vi "rad_Retrieve Application Image From Target.vi"(7 "App Images Temp Folder":path=path "C:/dev/Architectures/Reference Designs/Application Deployment and Replication/Application Deployment Utility/trunk/source/Application Images/_temp", 8 "error in (no error)":errorcluster, 10 "Target settings":T1={"Hostname"="", "Serial number"="", "Product name"="", "Product code"=0, "System status"="", "Credential type"=enum."None/Unlocked", "User added?"=FALSE, "Primary NIC"={"MAC address"="", "IP Address Request Mode"=2, "IP address"="", "Subnet mask"="", "Gateway"="", "DNS server"=""}} {"Primary NIC"."IP Address Request Mode" items=["Static"=1, "DHCP/Link-Local"=2, "Link-Local Only"=4, "DHCP Only"=8]}, 11 "App Images Folder":path) -> (0 "error out":errorcluster, 2 "Cancelled":bool, 3 "New App Image Path":path)   [LabVIEW 2014]
uses:
  TypeDefs/rad_Application Image Properties.ctl
  TypeDefs/rad_FPGA Properties.ctl
  TypeDefs/rad_FPGA Flash Properties.ctl
  Targets/TypeDefs/rad_Target Information.ctl
  Targets/TypeDefs/rad_Target Network Settings.ctl
  TypeDefs/rad_Retrieve Application Image States.ctl
  TypeDefs/rad_App Images Settings.ctl
  TypeDefs/rad_Deployment Status Data Type.ctl
  TypeDefs/rad_Deployment Progress Data Type.ctl
  TypeDefs/rad_Deployment Notifiers.ctl
panel:
  in  "State Data":T6
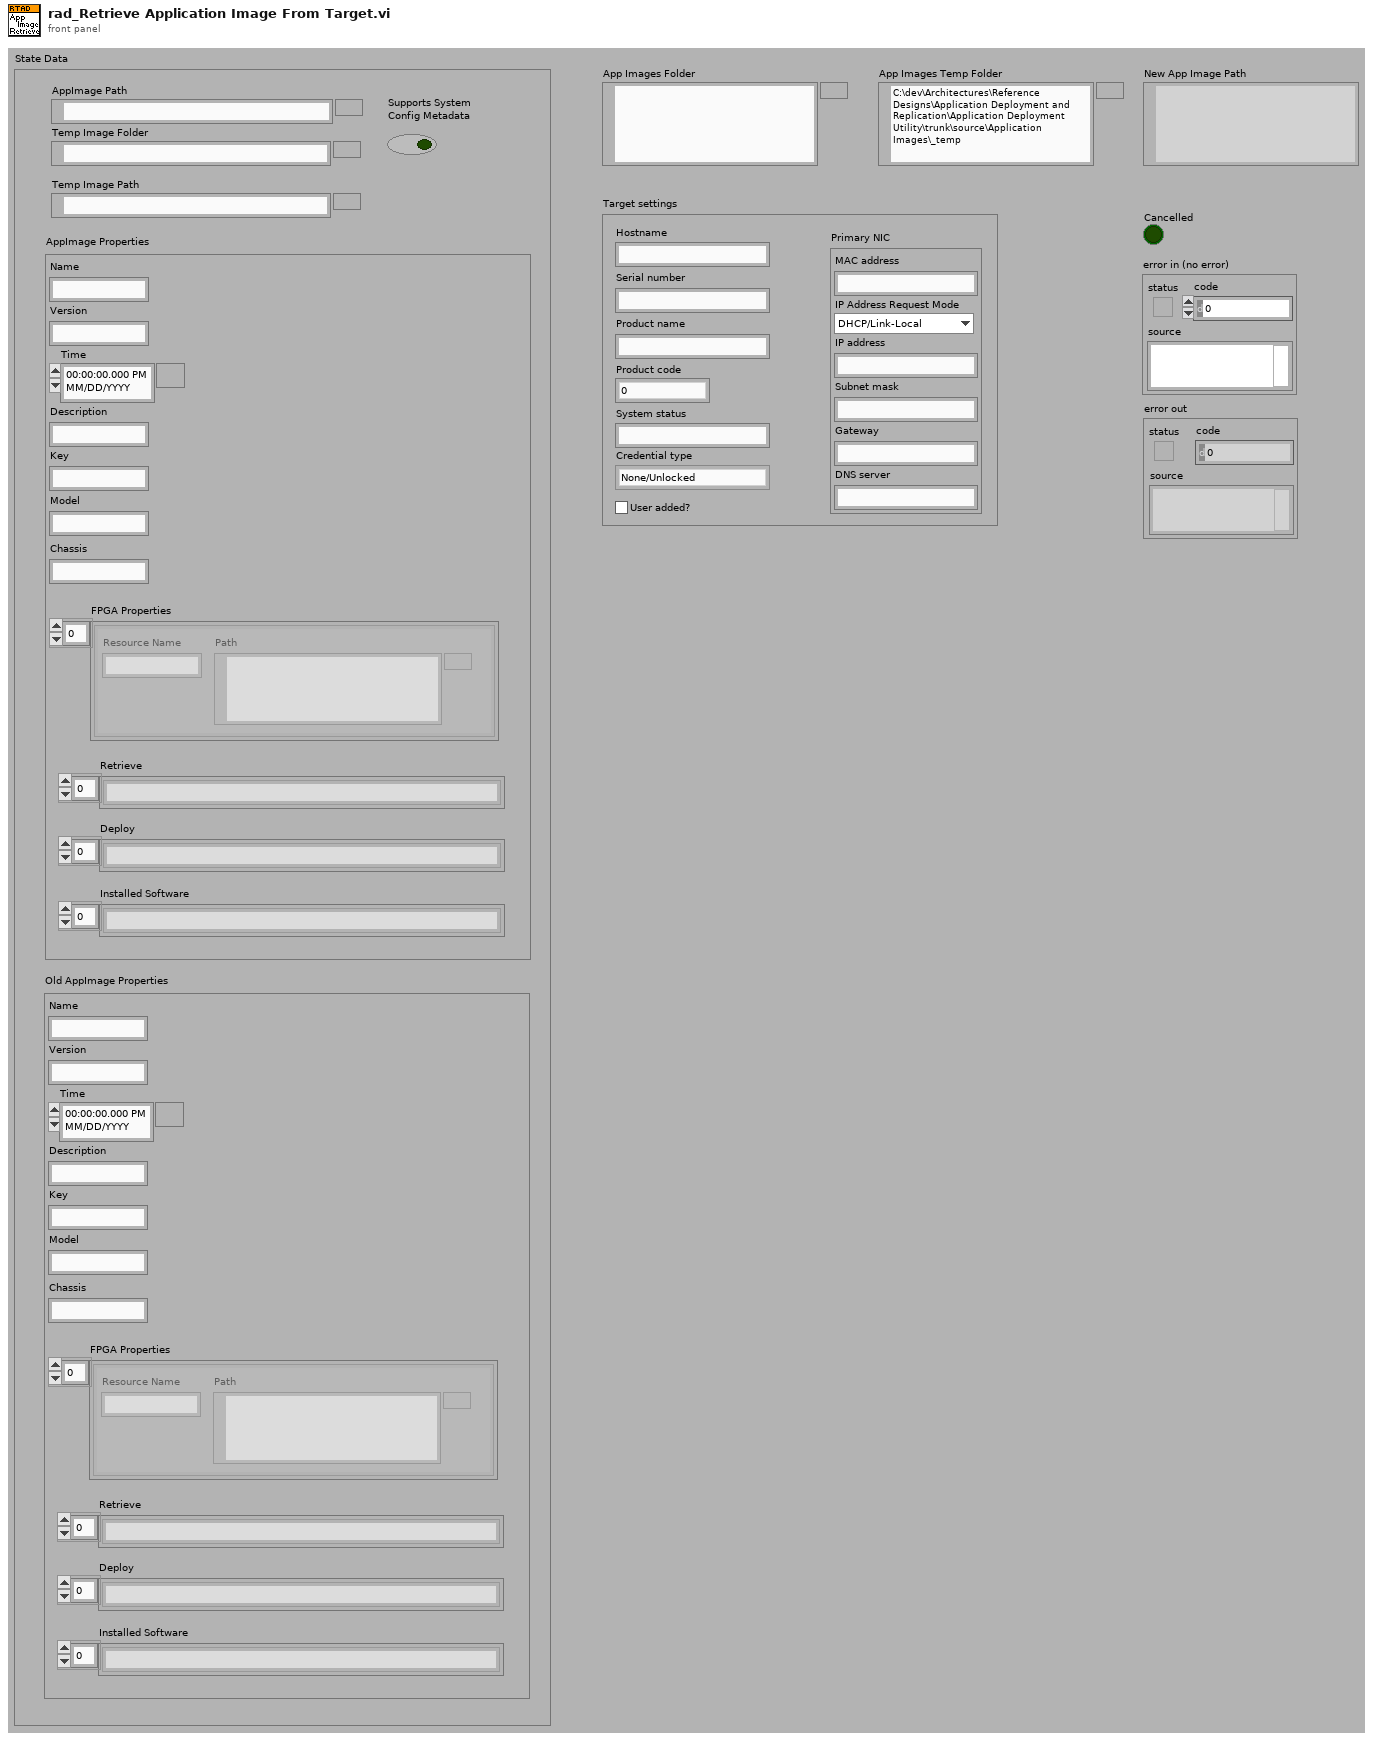
[diagram p1: front panel]
types:
  T1 = typedef "rad_Target Information.ctl" = cluster{"Hostname":string, "Serial number":string, "Product name":string, "Product code":i32, "System status":string, "Credential type":enum16{"None/Unlocked", "FTP Password", "NIAuth Credentials"}, "User added?":bool, "Primary NIC":T2}
  T2 = typedef "rad_Target Network Settings.ctl" = cluster{"MAC address":string, "IP Address Request Mode":i32, "IP address":string, "Subnet mask":string, "Gateway":string, "DNS server":string}
  T3 = typedef "rad_Application Image Properties.ctl" = cluster{"Name":string, "Version":string, "Time":timestamp, "Description":string, "Key":string, "Chassis":string, "FPGA Properties":T4, "Model":string, "Retrieve":string[], "Deploy":string[], "Installed Software":string[]}
  T4 = typedef "rad_FPGA Properties.ctl" = T5[]
  T5 = typedef "rad_FPGA Flash Properties.ctl" = cluster{"Resource Name":string, "Path":path}
  T6 = cluster{"AppImage Path":path, "Temp Image Folder":path, "AppImage Properties":T3, "App Image Info File Path":path, "New Image?":bool, "Selected Existing Image":path, "Bitfiles Modified?":bool, "Old AppImage Properties":T3, "Temp Image Path":path, "Supports System\nConfig Metadata":bool}
  T7 = typedef "rad_Retrieve Application Image States.ctl" = enum16{"Verify App Image Directory", "Get Target's Image Info", "Select Image Prop. Source", "Find Existing Disk Image", "Get Disk Image Properties", "Create New Image", "Set Image Properties", "Get Image Save Location", "GetInstalledSoftware", "Create App Image Info File", "Deploy New Files to Target", "Retrieve Application Image", "PackageImage", "Cleanup", "Exit"}
  T8 = typedef "rad_App Images Settings.ctl" = cluster{"App Images Folder":path, "App Images Temp Folder":path, "CurrentVersion":string}
  T9 = enum16{"None/Unlocked", "FTP Password", "NIAuth Credentials"}
  T10 = typedef "rad_Deployment Notifiers.ctl" = cluster{"Status":refnum<notifier>, "Progress":refnum<notifier>}
  T11 = typedef "rad_Deployment Progress Data Type.ctl" = i8
  T12 = typedef "rad_Deployment Status Data Type.ctl" = string
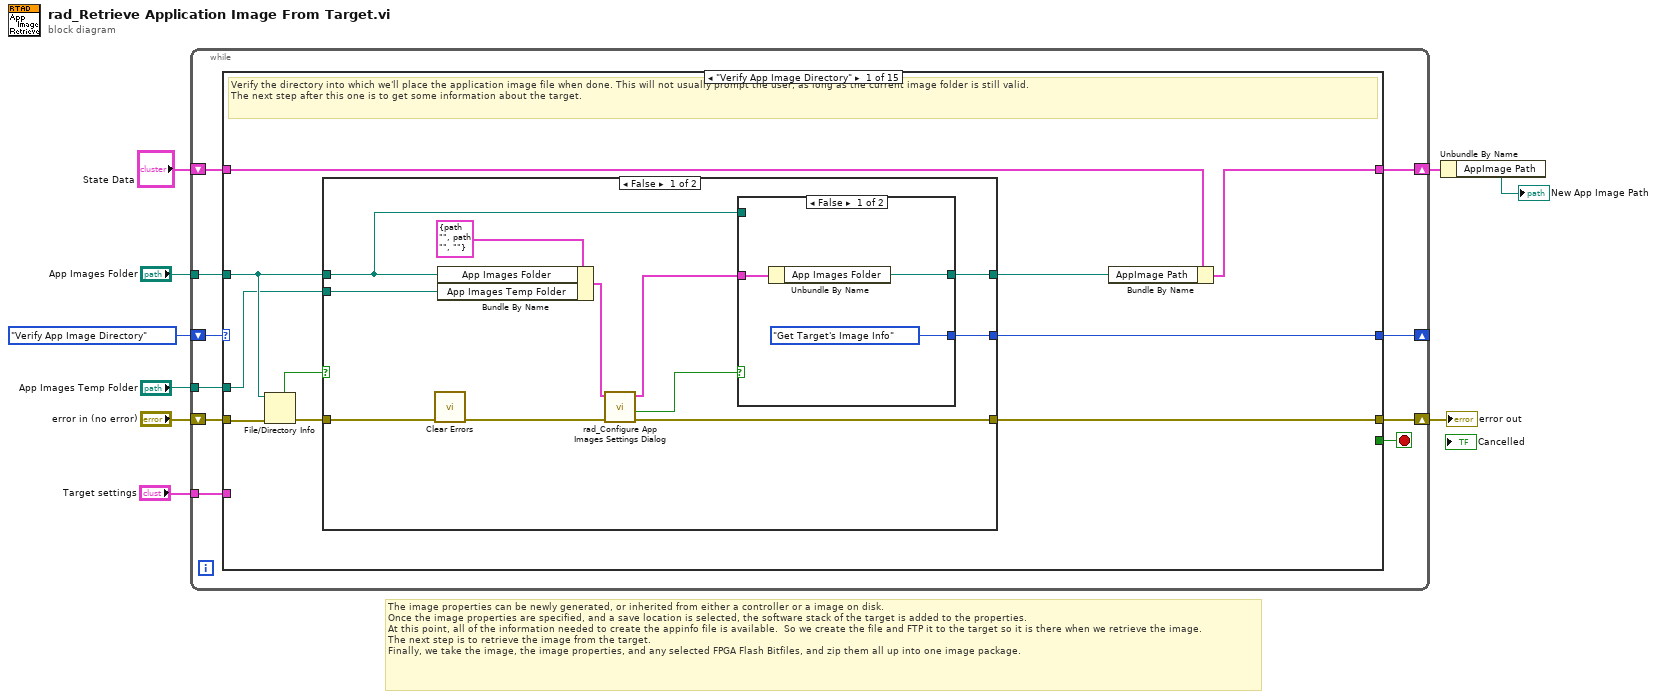
[diagram p0: block diagram]
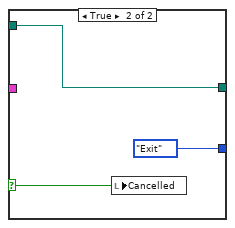
[diagram p2: hidden frame]
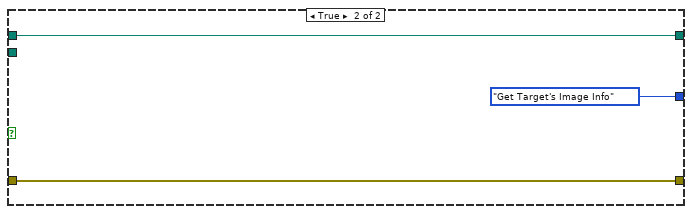
[diagram p3: hidden frame]
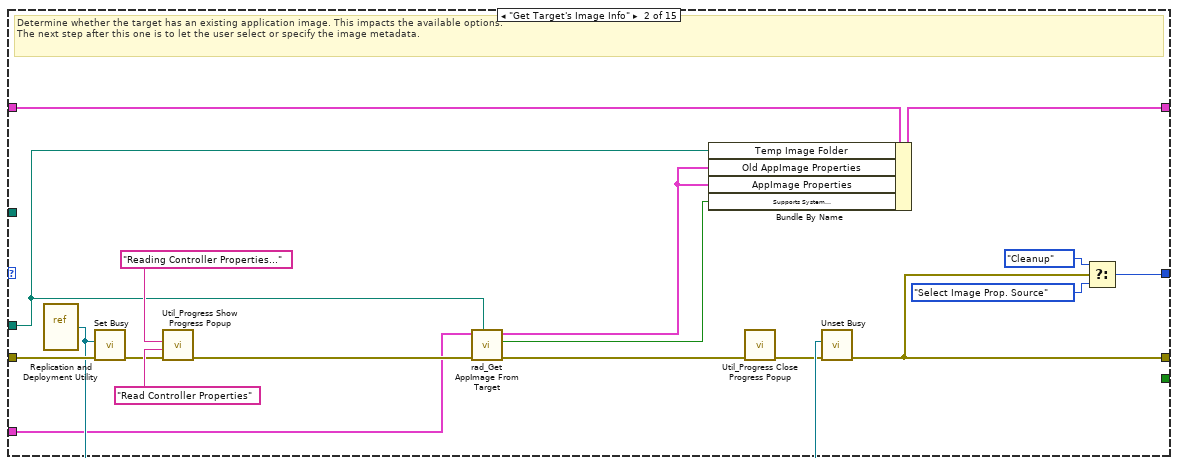
[diagram p4: hidden frame]
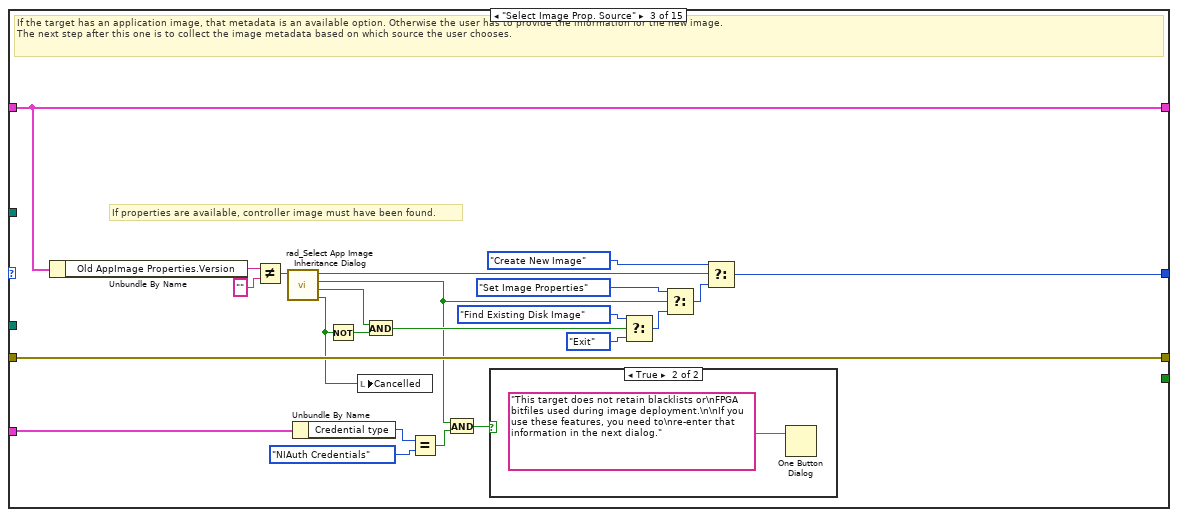
[diagram p5: hidden frame]
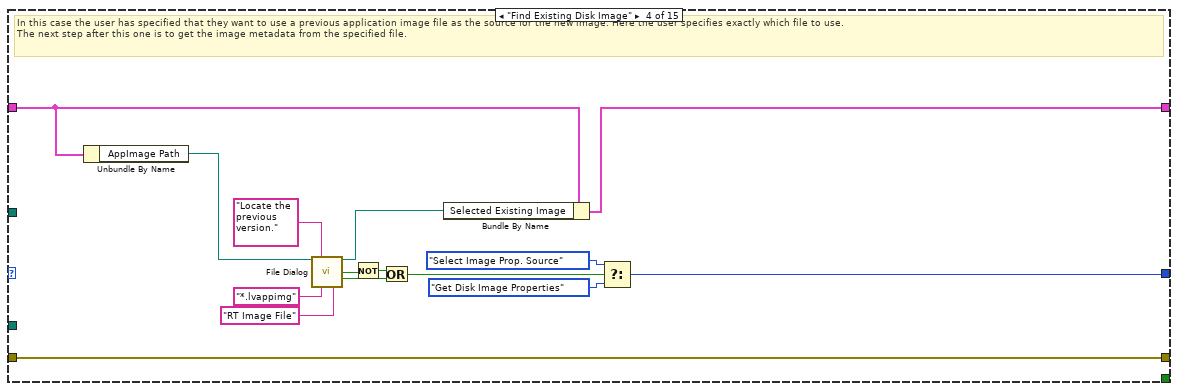
[diagram p7: hidden frame]
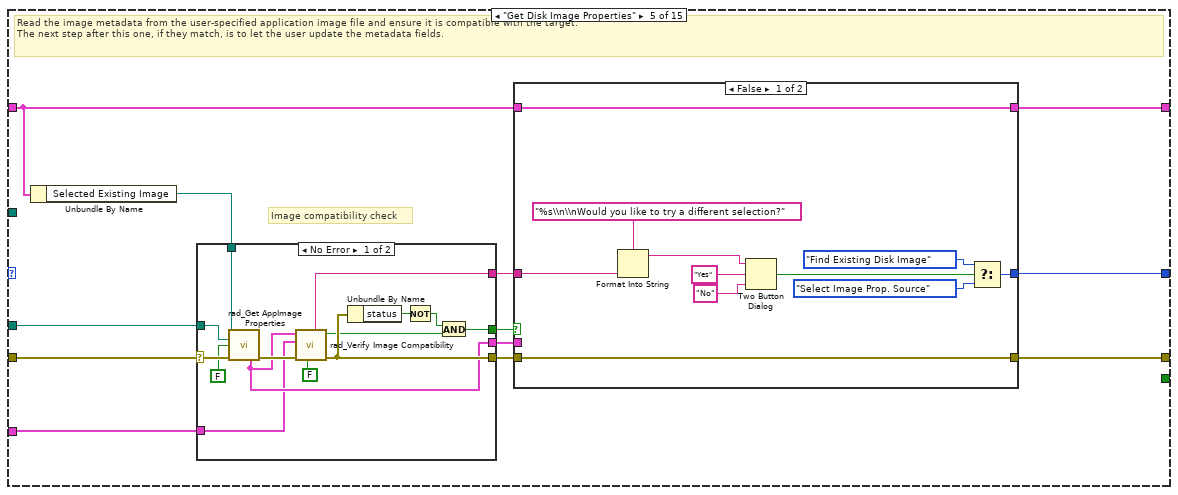
[diagram p8: hidden frame]
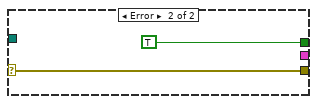
[diagram p9: hidden frame]
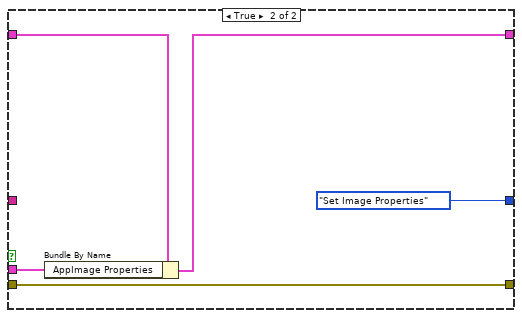
[diagram p10: hidden frame]
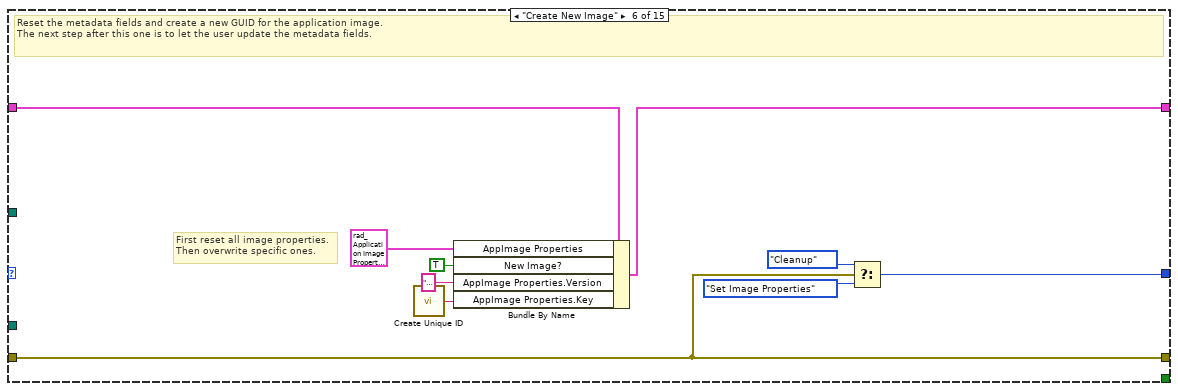
[diagram p11: hidden frame]
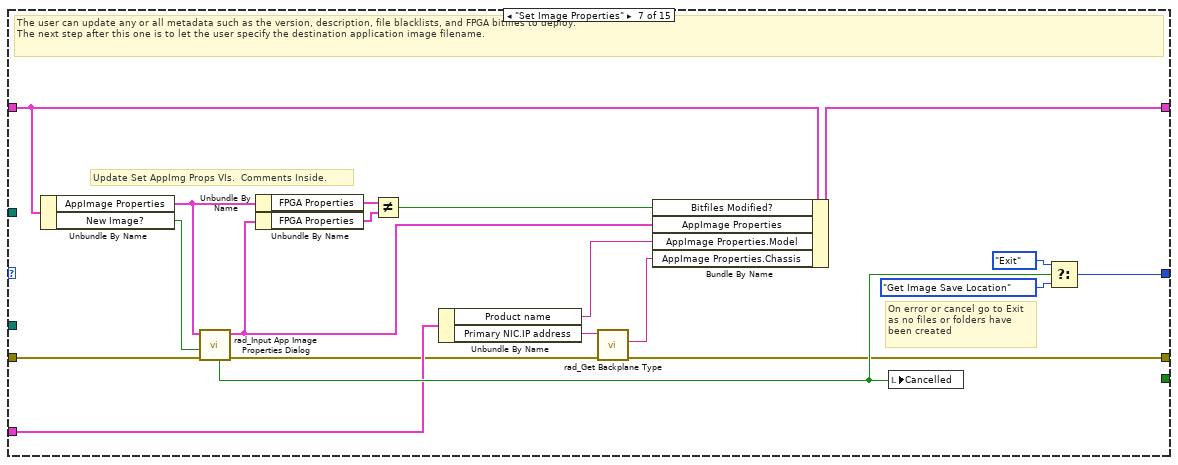
[diagram p12: hidden frame]
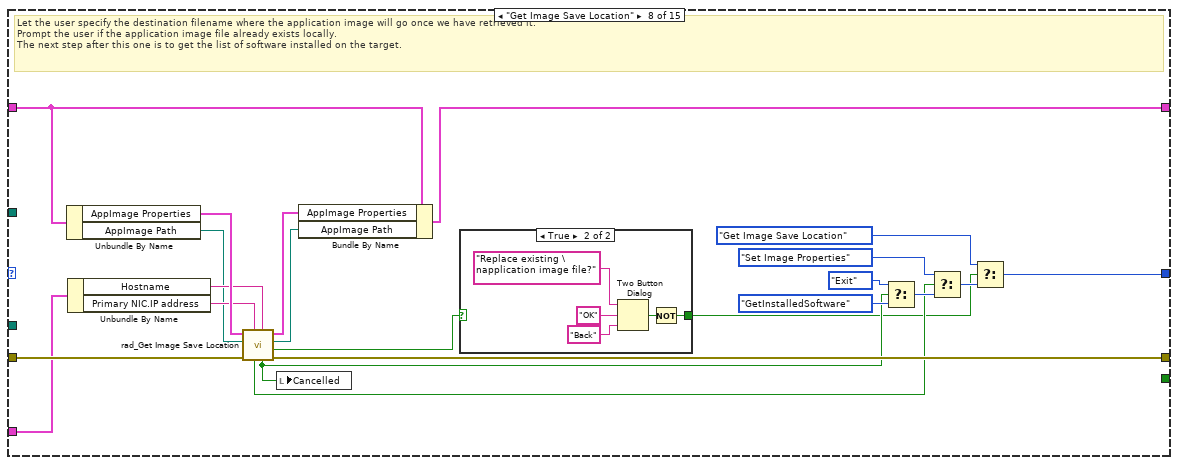
[diagram p13: hidden frame]
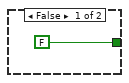
[diagram p14: hidden frame]
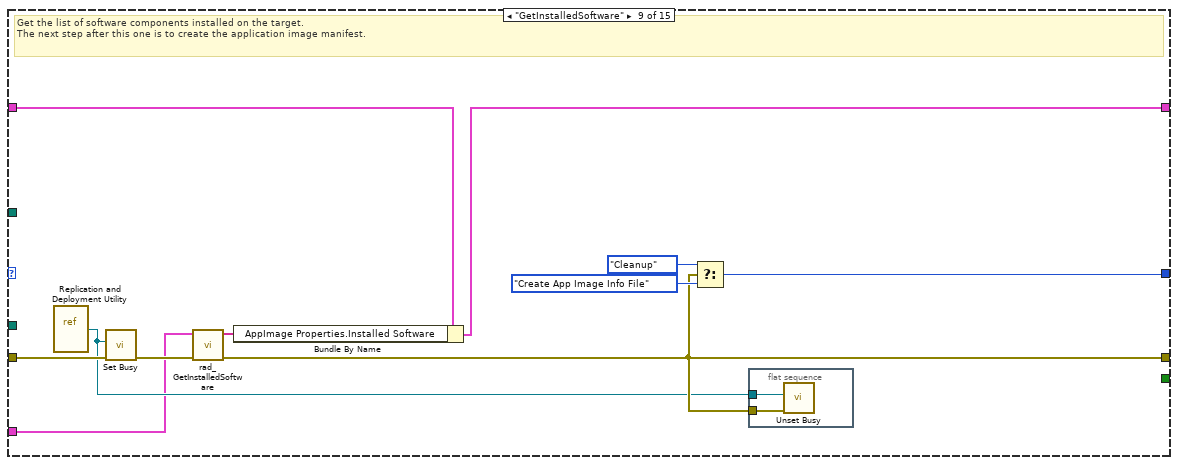
[diagram p15: hidden frame]
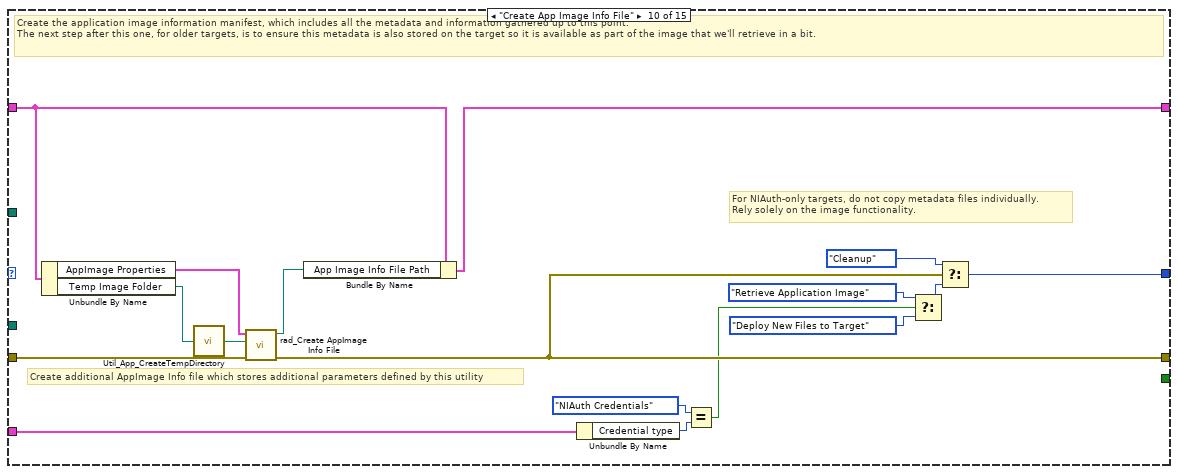
[diagram p16: hidden frame]
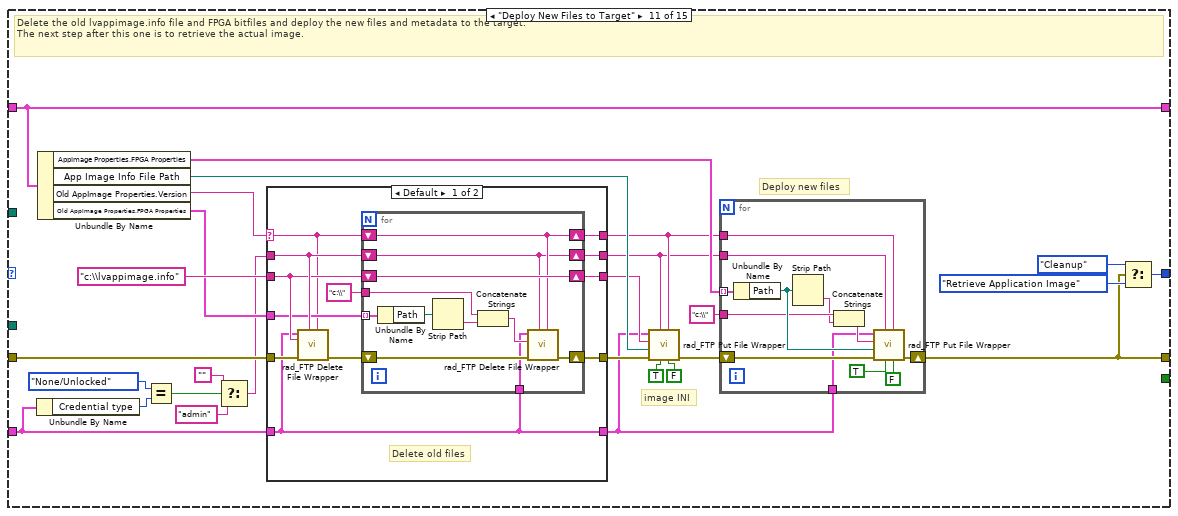
[diagram p17: hidden frame]
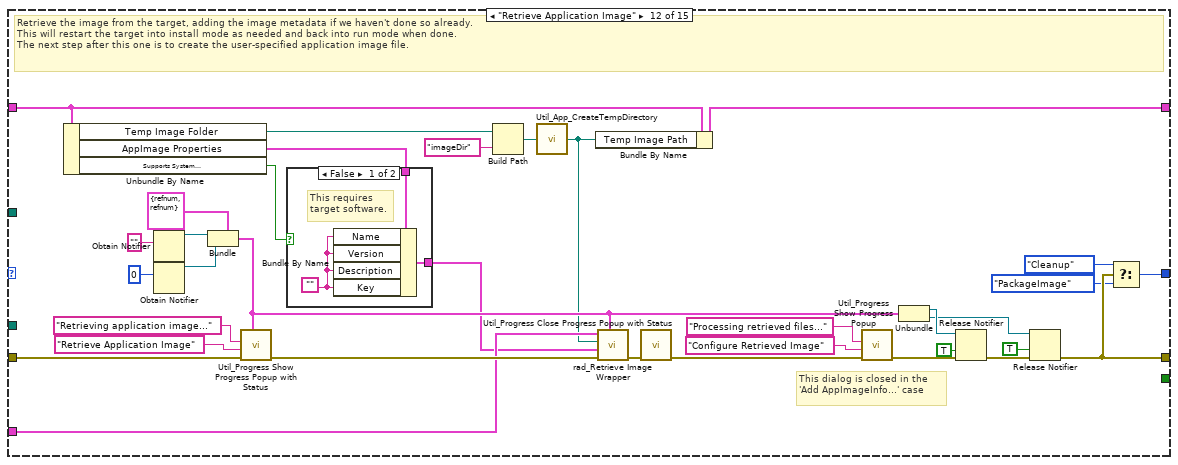
[diagram p19: hidden frame]
diagram:
  # "The image properties can be newly generated, or inherited from either a controller or a image on disk.\nOnce the image properties are specified, and a save location is selected, the software stack of the target is added to the properties.\nAt this point, all of the information needed to create the appinfo file is available.  So we create the file and FTP it to the target so it is there when we retrieve the image.\nThe next step is to retrieve the image from the target.\nFinally, we take the image, the image properties, and any selected FPGA Flash Bitfiles, and zip them all up into one image package."
  n1 = while {
    shift-right: [w18] -> _
    shift-left: rad_Retrieve_Application_Image_States."Verify App Image Directory" ("Retrieve App Images States") -> [w19]
    shift-right: [w15] -> w5
    shift-left: "State Data" -> [w16]
    shift-right: [w13] -> w6
    shift-left: "error in (no error)" -> [w14]
    tunnel: "App Images Folder" -> [w12]
    tunnel: "App Images Temp Folder" -> [w11]
    tunnel: "Target settings" -> [w10]
    stop <- w17 stop-if-true
    n2 = case shown="\"Verify App Image Directory\"" w19 {
      tunnel: [w23 w66 w78 w105 w117 w157 w179 w185 w214 w237 w249 w337 rad_Retrieve_Application_Image_States."Cleanup" ("Retrieve App Images States") rad_Retrieve_Application_Image_States."Exit" ("Retrieve App Images States") _] -> w18
      tunnel: [_ _ _ _ _ _ _ _ _ _ _ _ _ _ TRUE] -> w17
      tunnel: w16 -> [w22 w61 w90 w93 w114 w153 w174 w199 w217 w232 w264 w335 w347 w357 w371]
      tunnel: [w21 w65 w90 w104 w110 w160 w175 w198 w216 w234 w264 w336 w347 w357 w371] -> w15
      tunnel: w14 -> [w29 w60 w79 w106 w116 w151 w178 w201 w211 w230 w254 w330 w349 w351 w374]
      tunnel: [w26 w58 w79 w106 w112 w151 w161 w194 w212 w235 w248 w318 w348 w353 w374] -> w13
      tunnel: w12 -> [w25 _ _ _ _ _ _ _ _ _ _ _ _ _ _]
      tunnel: w11 -> [w24 w51 _ _ w111 _ _ _ _ _ _ _ _ _ _]
      tunnel: w10 -> [_ w52 w73 _ w107 _ w163 w183 w208 w224 w245 w311 _ _ _]
      frame "Verify App Image Directory" {
        # "Verify the directory into which we'll place the application image file when done. This will not usually prompt the user, as long as the current image folder is still valid.\nThe next step after this one is to get some information about the target."
        n3 = File/Directory Info(path=w25, error in=w29) -> (directory=w28:bool, error out=w27:errorcluster)  [unwired: 5 out]
        n4 = case shown="False" w28 {
          tunnel: w27 -> [w40 w49]
          tunnel: [w38 w49] -> w26
          tunnel: w25 -> [w30 w47]
          tunnel: w24 -> [w39 _]
          tunnel: [w35 rad_Retrieve_Application_Image_States."Get Target's Image Info" ("Retrieve App Images States")] -> w23
          tunnel: [w31 w47] -> w20
          frame False {
            n5 = call <vilib>:"Clear Errors.vi"("error in (no error)"=w40) -> ("error out"=w32:errorcluster)  [unwired: 5 in, 1 out]
            n6 = Bundle By Name(cluster=T8 {"App Images Folder"=path "", "App Images Temp Folder"=path "", "CurrentVersion"=""} ("App Images Settings"), "App Images Folder"=w30, "App Images Temp Folder"=w39) -> (w33:T8)
            n7 = call "rad_Configure App Images Settings Dialog.vi"("error in (no error)"=w32, "App Images Settings"=w33) -> ("error out"=w38:errorcluster, "Cancelled"=w37:bool, "App Images Settings"=w36:T8)  [unwired: 7 out]
            n8 = case shown="False" w37 {
              selector: w37 -> [_ w44]
              tunnel: w36 -> [w42 _]
              tunnel: [rad_Retrieve_Application_Image_States."Get Target's Image Info" ("Retrieve App Images States") rad_Retrieve_Application_Image_States."Exit" ("Retrieve App Images States")] -> w35
              tunnel: [w41 w45] -> w31
              tunnel: w30 -> [_ w45]
              frame False {
                n9 = Unbundle By Name(w42) -> ("App Images Folder"=w41:path)
              }
              frame True {
                n10 = local write "Cancelled"(w44) -> ()
              }
            }
          }
          frame True {
          }
        }
        n11 = Bundle By Name(cluster=w22, "AppImage Path"=w20) -> (w21:T6)
      }
      frame "Get Target's Image Info" {
        # "Determine whether the target has an existing application image. This impacts the available options.\nThe next step after this one is to let the user select or specify the image metadata."
        n12 = vi-ref "Replication and Deployment Utility.vi"() -> (w57:refnum<vi>)
        n13 = call <vilib>:"Set Busy.vi"("error in (no error)"=w60, "VI reference (current VI)"=w57) -> ("error out"=w59:errorcluster)  [unwired: 8 in, 1 out]
        n14 = call "Util_Progress Show Progress Popup.vi"("error in (no error)"=w59, "Title"="Read Controller Properties", "Message"="Reading Controller Properties...") -> ("error out"=w55:errorcluster)  [unwired: 8 in]
        n15 = call "rad_Get AppImage From Target.vi"("Temp Folder"=w51, "error in (no error)"=w55, "Target settings"=w52) -> ("error out"=w54:errorcluster, "Supports System\nConfig Metadata"=w50:bool, "AppImage Properties"=w53:T3)  [unwired: 6 in]
        n16 = Bundle By Name(cluster=w61, "Temp Image Folder"=w51, "Old AppImage Properties"=w53, "AppImage Properties"=w53, "Supports System\nConfig Metadata"=w50) -> (w65:T6)
        n17 = call "Util_Progress Close Progress Popup.vi"("error in (no error)"=w54) -> ("error out"=w56:errorcluster)  [unwired: 10 in]
        n18 = call <vilib>:"Unset Busy.vi"("error in (no error)"=w56, "VI reference (current VI)"=w57) -> ("error out"=w58:errorcluster)  [unwired: 9 in]
        n19 = Select(t=rad_Retrieve_Application_Image_States."Cleanup", s=w58, f=rad_Retrieve_Application_Image_States."Select Image Prop. Source" ("Retrieve App Images States")) -> (s? t:f=w66:T7)
      }
      frame "Select Image Prop. Source" {
        # "If properties are available, controller image must have been found."
        # "If the target has an application image, that metadata is an available option. Otherwise the user has to provide the information for the new image.\nThe next step after this one is to collect the image metadata based on which source the user chooses."
        n20 = Unbundle By Name(w90) -> ("Old AppImage Properties.Version"=w89:string)
        n21 = Not Equal?(x=w89, y="") -> (x != y?=w87:bool)
        n22 = call "rad_Select App Image Inheritance Dialog.vi"("Controller Image Available?"=w87) -> ("Cancel"=w74:bool, "Disc Image"=w77:bool, "Controller Image"=w69:bool, "New Image"=w86:bool)  [unwired: 7 in]
        n23 = Unbundle By Name(w73) -> ("Credential type"=w72:T9)
        n24 = Not(x=w74) -> (.not. x?=w76:bool)
        n25 = local write "Cancelled"(w74) -> ()
        n26 = And(x=w77, y=w76) -> (x .and. y?=w75:bool)
        n27 = Equal?(x=w72, y=T9."NIAuth Credentials" ("Credential type")) -> (x = y?=w70:bool)
        n28 = And(x=w69, y=w70) -> (x .and. y?=w68:bool)
        n29 = case shown="True" w68 {
          frame False {
          }
          frame True {
            n30 = One Button Dialog(message="This target does not retain blacklists or\nFPGA bitfiles used during image deployment.\n\nIf you use these features, you need to\nre-enter that information in the next dialog.") -> ()  [unwired: 1 in, 1 out]
          }
        }
        n31 = Select(t=rad_Retrieve_Application_Image_States."Find Existing Disk Image" ("Retrieve App Images States"), s=w75, f=rad_Retrieve_Application_Image_States."Exit" ("Retrieve App Images States")) -> (s? t:f=w81:T7)
        n32 = Select(t=rad_Retrieve_Application_Image_States."Set Image Properties" ("Retrieve App Images States"), s=w69, f=w81) -> (s? t:f=w83:T7)
        n33 = Select(t=rad_Retrieve_Application_Image_States."Create New Image" ("Retrieve App Images States"), s=w86, f=w83) -> (s? t:f=w78:T7)
      }
      frame "Find Existing Disk Image" {
        # "In this case the user has specified that they want to use a previous application image file as the source for the new image. Here the user specifies exactly which file to use.\nThe next step after this one is to get the image metadata from the specified file."
        n34 = Unbundle By Name(w93) -> ("AppImage Path"=w92:path)
        n35 = call "File Dialog"("start path"=w92, "prompt"="Locate the previous version.", "pattern (all files)"="*.lvappimg", "pattern label"="RT Image File") -> ("selected path"=w94:path, "exists"=w101:bool, "cancelled"=w99:bool)  [unwired: 8 in, 1 out]
        n36 = Not(x=w101) -> (.not. x?=w100:bool)
        n37 = Or(x=w100, y=w99) -> (x .or. y?=w97:bool)
        n38 = Bundle By Name(cluster=w93, "Selected Existing Image"=w94) -> (w104:T6)
        n39 = Select(t=rad_Retrieve_Application_Image_States."Select Image Prop. Source" ("f"), s=w97, f=rad_Retrieve_Application_Image_States."Get Disk Image Properties") -> (s? t:f=w105:T7)
      }
      frame "Get Disk Image Properties" {
        # "Image compatibility check"
        # "Read the image metadata from the user-specified application image file and ensure it is compatible with the target.\nThe next step after this one, if they match, is to let the user update the metadata fields."
        n40 = Unbundle By Name(w114) -> ("Selected Existing Image"=w118:path)
        n41 = case shown="No Error" w116 {
          selector: w116 -> [w124 w134]
          tunnel: w111 -> [w125 _]
          tunnel: w118 -> [w126 _]
          tunnel: [w132 w134] -> w113
          tunnel: [w130 TRUE] -> w115
          tunnel: [w121 _] -> w109
          tunnel: w107 -> [w120 _]
          tunnel: [w119 _] -> w108
          frame No Error {
            n42 = call "rad_Get AppImage Properties.vi"("AppImage Path"=w126, "App Image Temp Folder"=w125, "Show FP"=FALSE, "error in (no error)"=w124) -> ("AppImage Properties"=w121:T3, "error out"=w123:errorcluster)  [unwired: 5 in, 5 out]
            n43 = call "rad_Verify Image Compatibility.vi"("Require Identical Chassis?"=FALSE, "error in (no error)"=w123, "Target address"=w120, "AppImage Properties"=w121) -> ("error out"=w132:errorcluster, "Compatible?"=w129:bool, "Status message"=w119:string)  [unwired: 5 in]
            n44 = Unbundle By Name(w132) -> ("status"=w131:bool)
            n45 = Not(x=w131) -> (.not. x?=w128:bool)
            n46 = And(x=w128, y=w129) -> (x .and. y?=w130:bool)
          }
          frame Error {
          }
        }
        n47 = case shown="False" w115 {
          tunnel: [w140 rad_Retrieve_Application_Image_States."Set Image Properties" ("Retrieve App Images States")] -> w117
          tunnel: w114 -> [w138 w150]
          tunnel: w113 -> [w139 w146]
          tunnel: [w139 w146] -> w112
          tunnel: [w138 w148] -> w110
          tunnel: w109 -> [_ w147]
          tunnel: w108 -> [w136 _]
          frame False {
            n48 = Format Into String(format string="%s\\n\\nWould you like to try a different selection?" ("message"), w136) -> (resulting string=w135:string)  [unwired: 2 in, 1 out]
            n49 = Two Button Dialog(message=w135, 1:"No" ("F button name (\"Cancel\")"), 2:"Yes" ("T button name (\"OK\")")) -> (T button?=w142:bool)
            n50 = Select(t=rad_Retrieve_Application_Image_States."Find Existing Disk Image" ("Retrieve App Images States"), s=w142, f=rad_Retrieve_Application_Image_States."Select Image Prop. Source" ("Retrieve App Images States")) -> (s? t:f=w140:T7)
          }
          frame True {
            n51 = Bundle By Name(cluster=w150, "AppImage Properties"=w147) -> (w148:T6)
          }
        }
      }
      frame "Create New Image" {
        # "First reset all image properties.\nThen overwrite specific ones."
        # "Reset the metadata fields and create a new GUID for the application image.\nThe next step after this one is to let the user update the metadata fields."
        n52 = call "Create Unique ID.vi"() -> ("ID String"=w156:string)  [unwired: 1 in]
        n53 = Bundle By Name(cluster=w153, "AppImage Properties"=T3 {"Name"="", "Version"="", "Time"=timestamp(0 s since 1904-01-01), "Description"="", "Key"="", "Chassis"="", "FPGA Properties"=[], "Model"="", "Retrieve"=[], "Deploy"=[], "Installed Software"=[]}, "New Image?"=TRUE, "AppImage Properties.Version"="1.0.0", "AppImage Properties.Key"=w156) -> (w160:T6)
        n54 = Select(t=rad_Retrieve_Application_Image_States."Cleanup", s=w151, f=rad_Retrieve_Application_Image_States."Set Image Properties" ("Retrieve App Images States")) -> (s? t:f=w157:T7)
      }
      frame "Set Image Properties" {
        # "Update Set AppImg Props VIs.  Comments Inside."
        # "On error or cancel go to Exit\nas no files or folders have\nbeen created"
        # "The user can update any or all metadata such as the version, description, file blacklists, and FPGA bitfiles to deploy.\nThe next step after this one is to let the user specify the destination application image filename."
        n55 = Unbundle By Name(w174) -> ("AppImage Properties"=w169:T3, "New Image?"=w170:bool)
        n56 = call "rad_Input App Image Properties Dialog.vi"("error in (no error)"=w178, "New Image?"=w170, "AppImage Properties"=w169) -> ("error out"=w162:errorcluster, "AppImage Properties"=w167:T3, "Cancelled"=w168:bool)  [unwired: 4 in, 2 out]
        n57 = Unbundle By Name(w169) -> ("FPGA Properties"=w173:T4)
        n58 = Unbundle By Name(w167) -> ("FPGA Properties"=w172:T4)
        n59 = Not Equal?(x=w173, y=w172) -> (x != y?=w171:bool)
        n60 = Unbundle By Name(w163) -> ("Product name"=w165:string, "Primary NIC.IP address"=w166:string)
        n61 = call "rad_Get Backplane Type.vi"("error in (no error)"=w162, "Controller IP"=w166) -> ("error out"=w161:errorcluster, "Backplane Type"=w164:string)  [unwired: 7 in, 1 out]
        n62 = Bundle By Name(cluster=w174, "Bitfiles Modified?"=w171, "AppImage Properties"=w167, "AppImage Properties.Model"=w165, "AppImage Properties.Chassis"=w164) -> (w175:T6)
        n63 = local write "Cancelled"(w168) -> ()
        n64 = Select(t=rad_Retrieve_Application_Image_States."Exit" ("Retrieve App Images States"), s=w168, f=rad_Retrieve_Application_Image_States."Get Image Save Location" ("Retrieve App Images States")) -> (s? t:f=w179:T7)
      }
      frame "Get Image Save Location" {
        # "Let the user specify the destination filename where the application image will go once we have retrieved it.\nPrompt the user if the application image file already exists locally.\nThe next step after this one is to get the list of software installed on the target."
        n65 = Unbundle By Name(w199) -> ("AppImage Properties"=w200:T3, "AppImage Path"=w180:path)
        n66 = Unbundle By Name(w183) -> ("Hostname"=w182:string, "Primary NIC.IP address"=w181:string)
        n67 = call "rad_Get Image Save Location.vi"("Host Name"=w182, "IP Address"=w181, "error in (no error)"=w201, "Starting Path"=w180, "AppImage Properties"=w200) -> ("error out"=w194:errorcluster, "exists"=w195:bool, "Application Image Path"=w189:path, "AppImage Properties"=w197:T3, "Cancelled"=w188:bool, "Back"=w191:bool)  [unwired: 1 in]
        n68 = local write "Cancelled"(w188) -> ()
        n69 = Bundle By Name(cluster=w199, "AppImage Properties"=w197, "AppImage Path"=w189) -> (w198:T6)
        n70 = case shown="True" w195 {
          tunnel: [FALSE ("T button?") w203] -> w186
          frame False {
          }
          frame True {
            n71 = Two Button Dialog(message="Replace existing \napplication image file?", 1:"Back" ("F button name (\"Cancel\")"), 2:"OK" ("T button name (\"OK\")")) -> (T button?=w206:bool)
            n72 = Not(x=w206) -> (.not. x?=w203:bool)
          }
        }
        n73 = Select(t=rad_Retrieve_Application_Image_States."Exit" ("Retrieve App Images States"), s=w188, f=rad_Retrieve_Application_Image_States."GetInstalledSoftware" ("Retrieve App Images States")) -> (s? t:f=w192:T7)
        n74 = Select(t=rad_Retrieve_Application_Image_States."Set Image Properties", s=w191, f=w192) -> (s? t:f=w187:T7)
        n75 = Select(t=rad_Retrieve_Application_Image_States."Get Image Save Location", s=w186, f=w187) -> (s? t:f=w185:T7)
      }
      frame "GetInstalledSoftware" {
        # "Get the list of software components installed on the target.\nThe next step after this one is to create the application image manifest."
        n76 = vi-ref "Replication and Deployment Utility.vi"() -> (w209:refnum<vi>)
        n77 = call <vilib>:"Set Busy.vi"("error in (no error)"=w211, "VI reference (current VI)"=w209) -> ("error out"=w210:errorcluster)  [unwired: 8 in, 1 out]
        n78 = call "rad_GetInstalledSoftware.vi"("error in (no error)"=w210, "Target settings"=w208) -> ("error out"=w212:errorcluster, "installedSoftware"=w218:string[])  [unwired: 8 in]
        n79 = Bundle By Name(cluster=w217, "AppImage Properties.Installed Software"=w218) -> (w216:T6)
        n80 = Select(t=rad_Retrieve_Application_Image_States."Cleanup", s=w212, f=rad_Retrieve_Application_Image_States."Create App Image Info File" ("Retrieve App Images States")) -> (s? t:f=w214:T7)
        n81 = flat-sequence {
          tunnel: w212 -> [w220]
          tunnel: w209 -> [w219]
          frame #0 {
            n82 = call <vilib>:"Unset Busy.vi"("error in (no error)"=w220, "VI reference (current VI)"=w219) -> ()  [unwired: 9 in, 1 out]
          }
        }
      }
      frame "Create App Image Info File" {
        # "For NIAuth-only targets, do not copy metadata files individually.\nRely solely on the image functionality."
        # "Create additional AppImage Info file which stores additional parameters defined by this utility"
        # "Create the application image information manifest, which includes all the metadata and information gathered up to this point.\nThe next step after this one, for older targets, is to ensure this metadata is also stored on the target so it is available as part of the image that we'll retrieve in a bit."
        n83 = Unbundle By Name(w232) -> ("AppImage Properties"=w231:T3, "Temp Image Folder"=w221:path)
        n84 = call "Util_App_CreateTempDirectory.vi"("TempFolderPath"=w221) -> ("TempFolderPath_out"=w229:path)
        n85 = call "rad_Create AppImage Info File.vi"("error in (no error)"=w230, "Temp Image Folder"=w229, "AppImage Properties"=w231) -> ("error out"=w235:errorcluster, "App Image Info file path"=w233:path)  [unwired: 7 in]
        n86 = Bundle By Name(cluster=w232, "App Image Info File Path"=w233) -> (w234:T6)
        n87 = Unbundle By Name(w224) -> ("Credential type"=w226:T9)
        n88 = Equal?(x=T9."NIAuth Credentials" ("Credential type"), y=w226) -> (x = y?=w223:bool)
        n89 = Select(t=rad_Retrieve_Application_Image_States."Retrieve Application Image" ("Retrieve App Images States"), s=w223, f=rad_Retrieve_Application_Image_States."Deploy New Files to Target" ("Retrieve App Images States")) -> (s? t:f=w228:T7)
        n90 = Select(t=rad_Retrieve_Application_Image_States."Cleanup" ("Retrieve App Images States"), s=w235, f=w228) -> (s? t:f=w237:T7)
      }
      frame "Deploy New Files to Target" {
        # "Deploy new files"
        # "image INI"
        # "Delete the old lvappimage.info file and FPGA bitfiles and deploy the new files and metadata to the target.\nThe next step after this one is to retrieve the actual image."
        n91 = Unbundle By Name(w245) -> ("Credential type"=w243:T9)
        n92 = Unbundle By Name(w264) -> ("AppImage Properties.FPGA Properties"=w260:T4, "App Image Info File Path"=w263:path, "Old AppImage Properties.Version"=w238:string, "Old AppImage Properties.FPGA Properties"=w247:T4)
        n93 = Equal?(x=T9."None/Unlocked" ("Credential type"), y=w243) -> (x = y?=w241:bool)
        n94 = Select(t="", s=w241, f="admin" ("user")) -> (s? t:f=w246:string)
        n95 = case shown="Default" w238 {
          selector: w238 -> [w265 w288]
          tunnel: [w275 w288] -> w258
          tunnel: w246 -> [w274 w292]
          tunnel: [w273 w292] -> w257
          tunnel: "c:\\lvappimage.info" ("remote path") -> [w271 w291]
          tunnel: [w272 w291] -> w255
          tunnel: w254 -> [w276 w290]
          tunnel: [w267 w290] -> w253
          tunnel: w247 -> [w269 _]
          tunnel: w245 -> [w266 w289]
          tunnel: [w266 w289] -> w244
          frame Default {
            # "Delete old files"
            n96 = call "rad_FTP Delete File Wrapper.vi"("password"=w265, "user (admin)"=w274, "error in (no error)"=w276, "remote path"=w271, "Target settings"=w266) -> ("error out"=w268:errorcluster)  [unwired: 6 in]
            n97 = for {
              shift-right: [w282] -> w267
              shift-left: w268 -> [w281]
              tunnel: w269 -> [w287] mode=indexing
              tunnel: "c:\\" ("remote path") -> [w285]
              shift-right: [w279] -> w275
              shift-left: w265 -> [w279]
              shift-right: [w278] -> w273
              shift-left: w274 -> [w278]
              shift-right: [w283] -> w272
              shift-left: w271 -> [w283]
              tunnel: w266 -> [w277]
              n98 = Unbundle By Name(w287) -> ("Path"=w286:path)
              n99 = Strip Path(path=w286) -> (name=w284:string)  [unwired: 1 out]
              n100 = Concatenate Strings(w285, w284) -> (w280:string)
              n101 = call "rad_FTP Delete File Wrapper.vi"("password"=w279, "user (admin)"=w278, "error in (no error)"=w281, "remote path"=w280, "Target settings"=w277) -> ("error out"=w282:errorcluster)  [unwired: 6 in]
            }
          }
          frame "" {
          }
        }
        n102 = call "rad_FTP Put File Wrapper.vi"("active (F)"=FALSE ("active (T)"), "password"=w258, "binary (T)"=TRUE ("binary (F)"), "user (admin)"=w257, "error in (no error)"=w253, "local path"=w263, "remote path"=w255, "Target settings"=w244) -> ("error out"=w261:errorcluster)  [unwired: 3 in]
        n103 = for {
          shift-right: [w303] -> w248
          shift-left: w261 -> [w304]
          tunnel: w258 -> [w302]
          tunnel: w257 -> [w301]
          tunnel: w260 -> [w300] mode=indexing
          tunnel: "c:\\" ("remote path") -> [w298]
          tunnel: w244 -> [w293]
          n104 = Unbundle By Name(w300) -> ("Path"=w299:path)
          n105 = Strip Path(path=w299) -> (name=w297:string)  [unwired: 1 out]
          n106 = Concatenate Strings(w298, w297) -> (w296:string)
          n107 = call "rad_FTP Put File Wrapper.vi"("active (F)"=FALSE ("active (T)"), "password"=w302, "binary (T)"=TRUE ("binary (F)"), "user (admin)"=w301, "error in (no error)"=w304, "local path"=w299, "remote path"=w296, "Target settings"=w293) -> ("error out"=w303:errorcluster)  [unwired: 3 in]
        }
        n108 = Select(t=rad_Retrieve_Application_Image_States."Cleanup" ("Retrieve App Images States"), s=w248, f=rad_Retrieve_Application_Image_States."Retrieve Application Image" ("Retrieve App Images States")) -> (s? t:f=w249:T7)
      }
      frame "Retrieve Application Image" {
        # "This dialog is closed in the 'Add AppImageInfo...' case"
        # "Retrieve the image from the target, adding the image metadata if we haven't done so already.\nThis will restart the target into install mode as needed and back into run mode when done.\nThe next step after this one is to create the user-specified application image file."
        n109 = Unbundle By Name(w335) -> ("Temp Image Folder"=w308:path, "AppImage Properties"=w306:T3, "Supports System\nConfig Metadata"=w307:bool)
        n110 = Obtain Notifier(notification data type=T12 "" ("status notifier data type")) -> (notifier out=w323:refnum<notifier>)  [unwired: 3 in, 2 out]
        n111 = Obtain Notifier(notification data type=T11 0 ("Progress")) -> (notifier out=w324:refnum<notifier>)  [unwired: 3 in, 2 out]
        n112 = Bundle(cluster=T10 {"Status"=refnum, "Progress"=refnum} ("Deployment Notifiers"), "Status"=w323, "Progress"=w324) -> (w322:T10)
        n113 = call "Util_Progress Show Progress Popup with Status.vi"("Deployment Notifiers"=w322, "error in (no error)"=w330, "Title"="Retrieve Application Image", "Message"="Retrieving application image...") -> ("error out"=w329:errorcluster)  [unwired: 7 in]
        n114 = case shown="False" w307 {
          tunnel: w306 -> [w341 w342]
          tunnel: [w339 w342] -> w305
          frame False {
            w340 = ""
            # "This requires\ntarget software."
            n115 = Bundle By Name(cluster=w341, "Name"=w340, "Version"=w340, "Description"=w340, "Key"=w340) -> (w339:T3)
          }
          frame True {
          }
        }
        n116 = Build Path(base path=w308, name or relative path="imageDir") -> (appended path=w314:path)
        n117 = call "Util_App_CreateTempDirectory.vi"("TempFolderPath"=w314) -> ("TempFolderPath_out"=w309:path)
        n118 = Bundle By Name(cluster=w335, "Temp Image Path"=w309) -> (w336:T6)
        n119 = call "rad_Retrieve Image Wrapper.vi"("Deployment Notifiers"=w322, "error in (no error)"=w329, "AppImage Properties"=w305, "image file path"=w309, "Target settings"=w311) -> ("error out"=w313:errorcluster)  [unwired: 5 in, 1 out]
        n120 = call "Util_Progress Close Progress Popup with Status.vi"("error in (no error)"=w313) -> ("error out"=w326:errorcluster)  [unwired: 10 in]
        n121 = call "Util_Progress Show Progress Popup.vi"("error in (no error)"=w326, "Title"="Configure Retrieved Image", "Message"="Processing retrieved files...") -> ("error out"=w312:errorcluster)  [unwired: 8 in]
        n122 = Unbundle(w322) -> ("Status"=w321:refnum<notifier>, "Progress"=w320:refnum<notifier>)
        n123 = Release Notifier(notifier=w321, force destroy? (F)=TRUE, error in (no error)=w312) -> (error out=w319:errorcluster)  [unwired: 2 out]
        n124 = Release Notifier(notifier=w320, force destroy? (F)=TRUE, error in (no error)=w319) -> (error out=w318:errorcluster)  [unwired: 2 out]
        n125 = Select(t=rad_Retrieve_Application_Image_States."Cleanup" ("Retrieve App Images States"), s=w318, f=rad_Retrieve_Application_Image_States."PackageImage" ("Retrieve App Images States")) -> (s? t:f=w337:T7)
      }
      frame "PackageImage" {
        # "Incorporate the application manifest with the temporary image and other relevant files into the user-specified application image file.\nThe next step after this one is to start cleaning up."
        n126 = Unbundle By Name(w347) -> ("AppImage Properties.FPGA Properties"=w346:T4, "App Image Info File Path"=w345:path, "Temp Image Path"=w344:path, "AppImage Path"=w343:path)
        n127 = call "rad_PackageImage.vi"("AppImage Properties.FPGA Properties"=w346, "error in (no error)"=w349, "AppImage Path"=w343, "Temp Image Path"=w344, "App Image Info File Path"=w345) -> ("error out"=w348:errorcluster)  [unwired: 6 in]
      }
      frame "Cleanup" {
        # "We finished the image retrieval process, let the user know the final status.\nThe next step after this one is to finish cleaning up."
        n128 = call "Util_Progress Close Progress Popup.vi"("error in (no error)"=w351) -> ("error out"=w352:errorcluster)  [unwired: 10 in]
        n129 = Unbundle By Name(w352) -> ("code"=w355:i32, "source"=w356:string)
        n130 = case shown="0, 221" w355 {
          selector: w355 -> [_ _ w367]
          tunnel: w356 -> [_ _ w370]
          tunnel: ["Application image retrieval successful." ("source") "Error 56 Occurred: Unable to establish communication with the target.  Verify that your network settings are valid." ("source") w369] -> w354
          tunnel: [w359 w362 w365] -> w353
          tunnel: w352 -> [w360 w363 w366]
          frame 0, 221 {
            n131 = call <vilib>:"Clear Errors.vi"("error in (no error)"=w360) -> ("error out"=w359:errorcluster)  [unwired: 5 in, 1 out]
          }
          frame 56 {
            n132 = call <vilib>:"Clear Errors.vi"("error in (no error)"=w363) -> ("error out"=w362:errorcluster)  [unwired: 5 in, 1 out]
          }
          frame Default {
            n133 = Format Into String(format string="Application Image Retrieval Error:\\r\\n %s - %d", w370, w367) -> (resulting string=w369:string)  [unwired: 2 in, 1 out]
            n134 = call <vilib>:"Clear Errors.vi"("error in (no error)"=w366) -> ("error out"=w365:errorcluster)  [unwired: 5 in, 1 out]
          }
        }
        n135 = One Button Dialog(message=w354) -> ()  [unwired: 2 out]
      }
      frame "Exit" {
        # "Remove the temporary folder and all contents (including the temporary image) created in the various stages of this process.\nThis is the final step."
        n136 = Unbundle By Name(w371) -> ("Temp Image Folder"=w373:path)
        n137 = Delete(path (use dialog)=w373, entire hierarchy (F)=TRUE) -> ()  [unwired: 1 in, 5 out]
      }
    }
  }
  "error out" <- w6
  n138 = Unbundle By Name(w5) -> ("AppImage Path"=→"New App Image Path":path)
